vi "Read Inputs from system.vi"(8 "error in":errorcluster, 11 "DAQmx Watchdog runtime in":refnum<class "DAQmx Watchdog runtime.lvclass">) -> (0 "error out":errorcluster, 2 "Inputs from system":T1, 3 "DAQmx Watchdog runtime out":refnum<class "DAQmx Watchdog runtime.lvclass">)   [LabVIEW 2014, in "DAQmx Watchdog runtime.lvclass"]
uses:
  DAQmx Watchdog runtime.lvclass
  configuration/input data indices.ctl
  DAQmx Watchdog runtime.lvclass/DAQmx Watchdog runtime.ctl
  configuration/DAQmx Watchdog configuration.lvclass
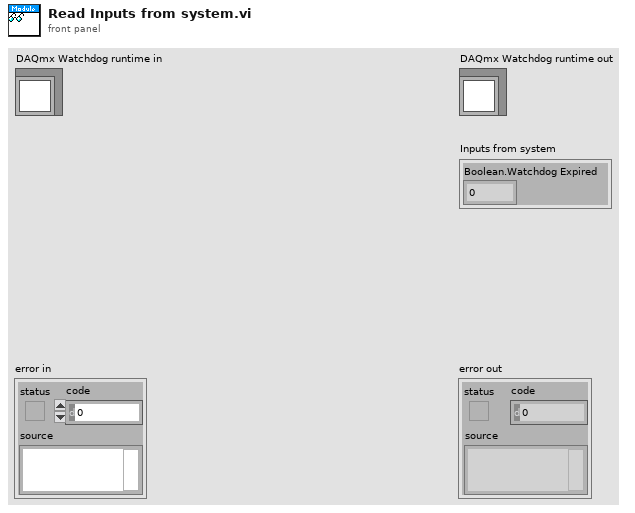
[diagram p1: front panel]
types:
  T1 = typedef "DAQmx Watchdog configuration.lvclass/input data indices.ctl" = cluster{"Boolean.Watchdog Expired":i32}
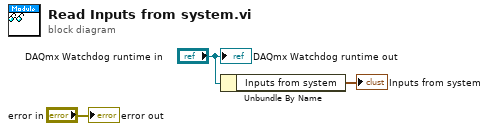
[diagram p0: block diagram]
diagram:
  n1 = Unbundle By Name("DAQmx Watchdog runtime in") -> ("Inputs from system"=→"Inputs from system":T1)
  "error out" <- "error in"
  "DAQmx Watchdog runtime out" <- "DAQmx Watchdog runtime in"
